vi "FireByName.vi"(8 "error in (no error)":errorcluster, 9 "Data":variant, 10 "Msg":string, 11 "object in":refnum<class "EventMsg.lvclass">) -> (0 "error out":errorcluster, 3 "object out":refnum<class "EventMsg.lvclass">)   [LabVIEW 2014, in "EventMsg.lvclass"]
doc: "Fire event Msg to the Named Event.\n\nIs possible to use Masg String to write a sequence steps in a spreadsheet format.\nMsg are like \nInit/nStore/n and so on"
uses:
  EventMsg.lvclass
  EventMsg.lvclass/EventMsg.ctl
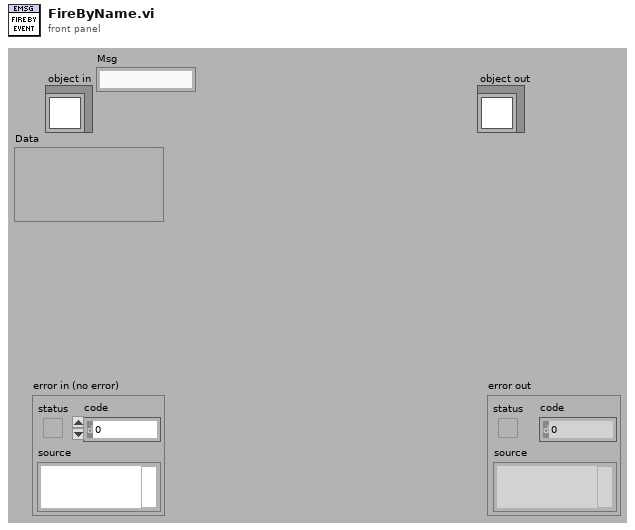
[diagram p1: front panel]
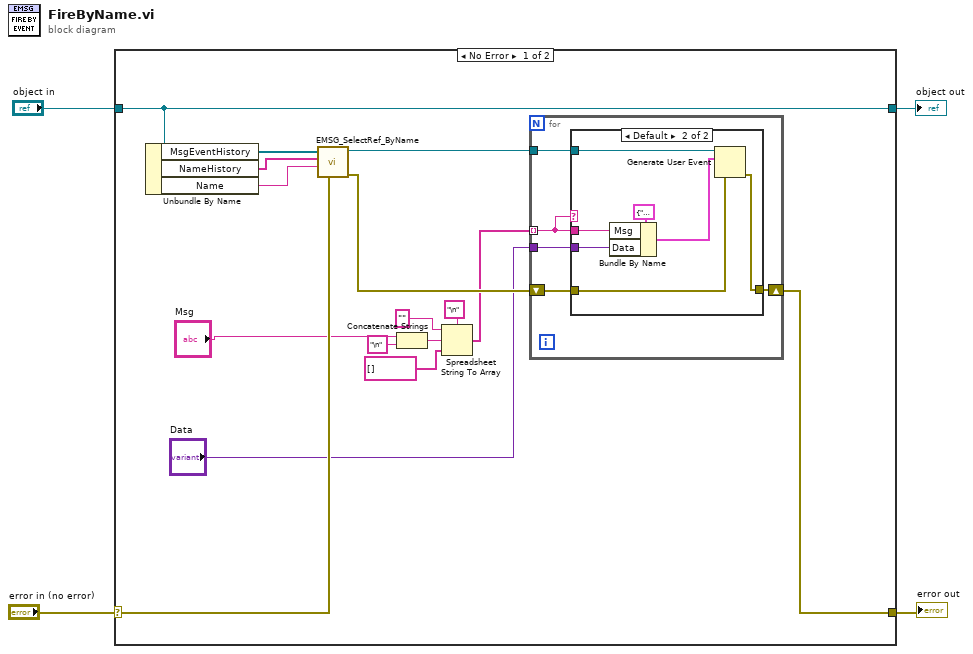
[diagram p0: block diagram]
diagram:
  n1 = case shown="No Error" "error in (no error)" {
    selector: "error in (no error)" -> [w15 w35]
    tunnel: [w19 w35] -> w3
    tunnel: [w20 w34] -> w1
    tunnel: "object in" -> [w20 w34]
    frame No Error {
      n2 = Unbundle By Name(w20) -> ("MsgEventHistory"=w18:refnum<user-event>[], "NameHistory"=w16:string[], "Name"=w5:string)
      n3 = call "EMSG_SelectRef_ByName.vi"("Error in"=w15, "Name"=w5, "NameHistory"=w16, "MsgEventHistory"=w18) -> ("Error out"=w14:errorcluster, "User Event out"=w17:refnum<user-event>)  [unwired: 6 in]
      n4 = Concatenate Strings("Msg", "\n" ("string")) -> (w9:string)
      n5 = Spreadsheet String To Array(delimiter (Tab)="\n", format string="", spreadsheet string=w9, array type (2D Dbl)=string[] []) -> (array=w10:string[])
      n6 = for {
        tunnel: w17 -> [w24]
        shift-right: [w25] -> w19
        shift-left: w14 -> [w23]
        tunnel: w10 -> [w21] mode=indexing
        tunnel: "Data" -> [w22]
        n7 = case shown="Default" w21 {
          tunnel: [w26 w33] -> w25
          tunnel: w24 -> [_ w32]
          tunnel: w23 -> [w26 w31]
          tunnel: w21 -> [_ w28]
          tunnel: w22 -> [_ w27]
          frame "\u0000" {
          }
          frame Default {
            n8 = Bundle By Name(cluster=cluster{"Msg":string, "Data":variant} {"Msg"="", "Data"=variant} ("event data"), "Msg"=w28, "Data"=w27) -> (w29:cluster{"Msg":string, "Data":variant})
            n9 = Generate User Event(user event=w32, event data cluster=w29, error in=w31) -> (error out=w33:errorcluster)  [unwired: 1 in, 1 out]
          }
        }
      }
    }
    frame Error {
    }
  }
  "error out" <- w3
  "object out" <- w1
